vi "Prompt for Overwrite.vi"(8 "error in (no error)":errorcluster, 11 "path":path) -> (0 "error out":errorcluster, 1 "Overwrite":bool, 2 "New File":bool, 3 "dup path":path)   [LabVIEW 2014]
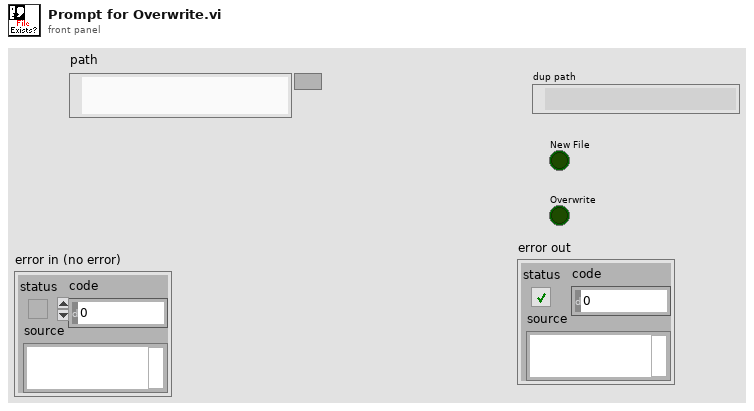
[diagram p1: front panel]
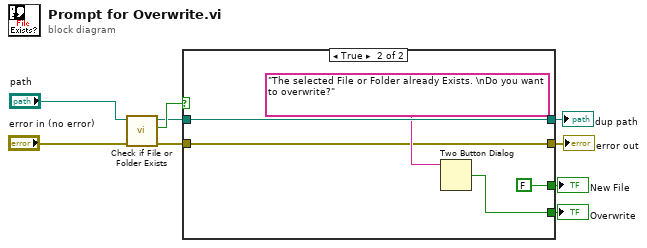
[diagram p0: block diagram]
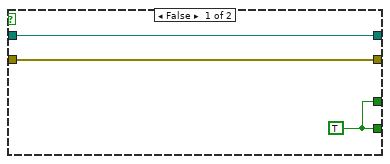
[diagram p2: hidden frame]
diagram:
  n1 = call <vilib>:"Check if File or Folder Exists.vi"("error in (no error)"="error in (no error)", "path"="path") -> ("error out"=w8:errorcluster, "file or folder exists?"=w9:bool, "dup path"=w7:path)  [unwired: 7 in]
  n2 = case shown="True" w9 {
    tunnel: w8 -> [w11 w14]
    tunnel: [w12 w17] -> w3
    tunnel: w7 -> [w12 w17]
    tunnel: [w11 w14] -> w2
    tunnel: [w10 w16] -> w4
    tunnel: [w10 FALSE] -> w1
    frame False {
      w10 = TRUE
    }
    frame True {
      n3 = Two Button Dialog(message="The selected File or Folder already Exists. \nDo you want to overwrite?") -> (T button?=w16:bool)  [unwired: 2 in]
    }
  }
  "Overwrite" <- w4
  "dup path" <- w3
  "error out" <- w2
  "New File" <- w1
